vi "dBm_to_ASF.vi"(1 "Amplitude (dBm)":dbl, 12 "Channel Parameters":T1 {"Ref Clock Rate [MHz]" min=0.0}) -> (21 "ASF":u32)   [LabVIEW 2013, in "DDS.lvlib"]
uses:
  DDS.lvlib
  Controls/DDS Channel Parameters.ctl
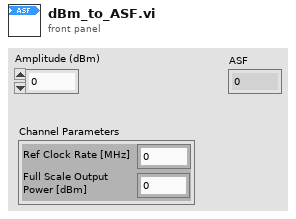
[diagram p1: front panel]
types:
  T1 = typedef "DDS.lvlib/DDS Channel Parameters.ctl" = cluster{"Ref Clock Rate [MHz]":dbl, "Full Scale Output\nPower [dBm]":dbl}
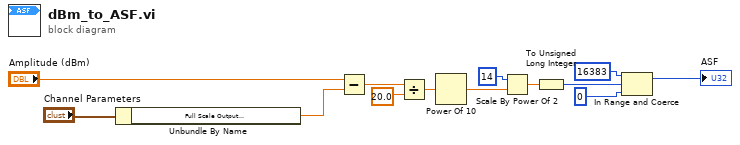
[diagram p0: block diagram]
diagram:
  n1 = Unbundle By Name("Channel Parameters") -> ("Full Scale Output\nPower [dBm]"=w1:dbl)
  n2 = Subtract(x="Amplitude (dBm)", y=w1) -> (x-y=w12:dbl)
  n3 = Divide(x=w12, y=20.0) -> (x/y=w10:dbl)
  n4 = Power Of 10(x=w10) -> (10^x=w9:dbl)
  n5 = Scale By Power Of 2(n=14, x=w9) -> (x*2^n=w7:dbl)
  n6 = To Unsigned Long Integer(number=w7) -> (unsigned 32bit integer=w4:u32)
  n7 = In Range and Coerce(upper limit=u32 16383, x=w4, lower limit=u32 0) -> (coerced(x)=→"ASF":u32)  [unwired: 1 out]
